vi "PH_DataViewer.set Powermeter GUI elements.vi"(2 "Powermeters":T1[](array[typedef]) {"Device State" items=["no info", "off/false", "on/true", "Failure", "Alarm"]}, 5 "Version":u8) -> (10 "Instances":string[](array[string]), 11 "Status":u32, 12 "index":i32, 13 "Trigger Level":dbl, 14 "Snapshot: Date":string, 15 "Snapshot: Time":string, 16 "Serial Number":string, 17 "Current Value":dbl, 18 "Current Value Unit":string, 19 "Scaling Factor":dbl)   [LabVIEW 2014, in "PH_DataViewer.lvlib"]
doc: "This VI prepares the information to be indicated."
uses:
  PH_DataViewer.lvlib
  PH_gentec_Powermeter.Data.ctl
  PH_DataViewer.Device State.ctl
  PH_Basics/PH_Common/PH_Common.lvlib
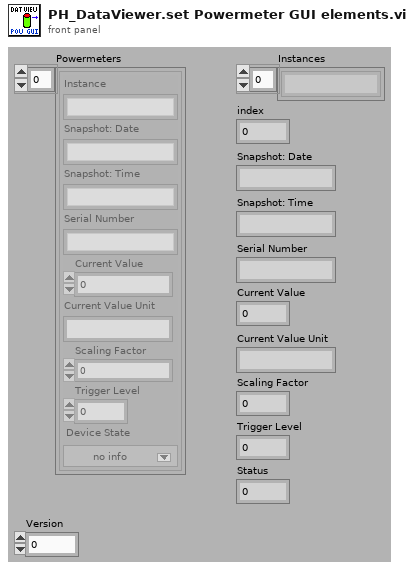
[diagram p1: front panel]
types:
  T1 = typedef "PH_DataViewer.lvlib/PH_gentec_Powermeter.Data.ctl" = cluster{"Instance":string, "Snapshot: Date":string, "Snapshot: Time":string, "Serial Number":string, "Current Value":dbl, "Current Value Unit":string, "Scaling Factor":dbl, "Trigger Level":dbl, "Device State":T2}
  T2 = typedef "PH_DataViewer.lvlib/PH_DataViewer.Device State.ctl" = i32
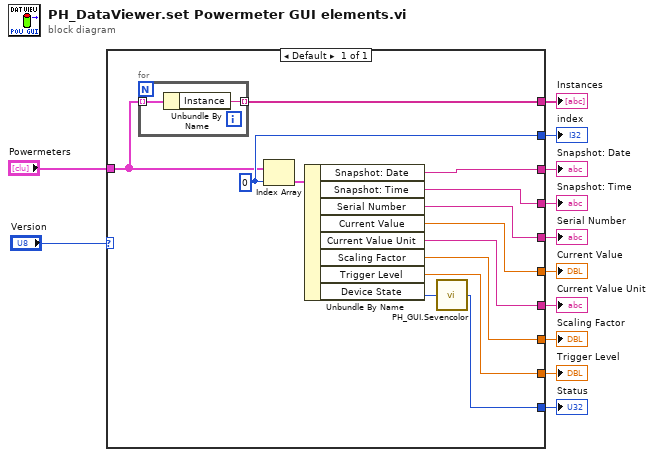
[diagram p0: block diagram]
diagram:
  n1 = case shown="Default" "Version" {
    tunnel: [w25] -> w12
    tunnel: [w23] -> w11
    tunnel: [w22] -> w10
    tunnel: "Powermeters" -> [w21]
    tunnel: [w20] -> w8
    tunnel: [w19] -> w7
    tunnel: [w18] -> w6
    tunnel: [w17] -> w5
    tunnel: [w16] -> w4
    tunnel: [w15] -> w3
    tunnel: [w14] -> w2
    frame Default {
      w23 = 0 ("index")
      n2 = for {
        tunnel: w21 -> [w27] mode=indexing
        tunnel: [w26] -> w22 mode=indexing
        n3 = Unbundle By Name(w27) -> ("Instance"=w26:string)
      }
      n4 = Index Array(array=w21, index=w23) -> (element=w13:T1)
      n5 = Unbundle By Name(w13) -> ("Snapshot: Date"=w15:string, "Snapshot: Time"=w14:string, "Serial Number"=w19:string, "Current Value"=w16:dbl, "Current Value Unit"=w20:string, "Scaling Factor"=w17:dbl, "Trigger Level"=w18:dbl, "Device State"=w24:T2)
      n6 = call "PH_GUI.Sevencolor.vi"("State"=w24) -> ("Color Box"=w25:u32)
    }
  }
  "Status" <- w12
  "index" <- w11
  "Instances" <- w10
  "Current Value Unit" <- w8
  "Serial Number" <- w7
  "Trigger Level" <- w6
  "Scaling Factor" <- w5
  "Current Value" <- w4
  "Snapshot: Date" <- w3
  "Snapshot: Time" <- w2
